vi "AbsU64.vi"(4 "x":u64) -> (1 "Abs(x)":u64, 2 "Overflow?":bool)   [LabVIEW 2017, in "GPOverflow.lvlib"]
doc: "Returns the absolute value of <B>x</B> keeping track of numeric overflow.\n\n<B>Overflow?</B> will be True if overflow occurred. The output will saturate in case of overflow.\n\nThis VI is inlined.\n\nSteen Schmidt\nGPower\n26/12 2013"
uses:
  GPOverflow.lvlib
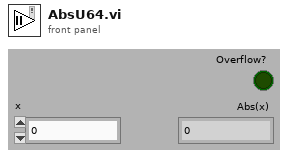
[diagram p1: front panel]
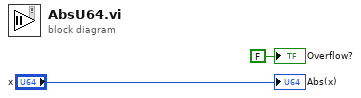
[diagram p0: block diagram]
diagram:
  "Abs(x)" <- "x"
  "Overflow?" <- FALSE ("Overflow?")
